vi "Printer Error Handler.vi"(8 "에러 입력(에러 없음)":errorcluster, 10 "큐 데이터":string, 11 "상태":T1 caption="상태 입력") -> (0 "에러 출력":errorcluster, 3 "다음 상태":T1)   [LabVIEW 2010]
doc: "이 템플릿을 사용하여 SubVI로 사용할 VI를 만듭니다."
uses:
  Print Processing States.ctl
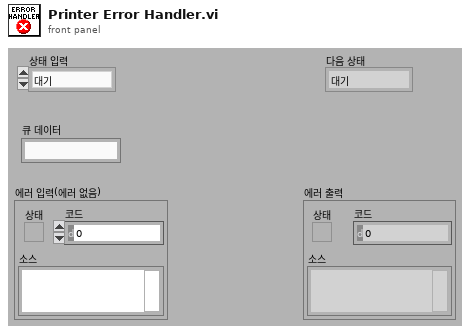
[diagram p1: front panel]
types:
  T1 = typedef "Print Processing States.ctl" = enum16{"대기", "셋업 초기화", "셋업", "인쇄 초기화", "인쇄", "종료"}
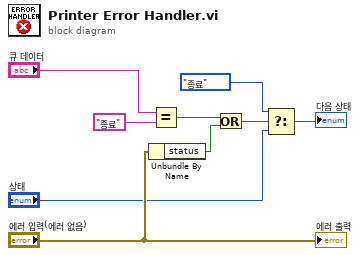
[diagram p0: block diagram]
diagram:
  n1 = Unbundle By Name("에러 입력(에러 없음)") -> ("status"=w6:bool)
  n2 = Equal?(x="큐 데이터", y="종료") -> (x = y?=w5:bool)
  n3 = Or(x=w5, y=w6) -> (x .or. y?=w4:bool)
  n4 = Select(t=Print_Processing_States."종료", s=w4, f="상태") -> (s? t:f=→"다음 상태":T1)
  "에러 출력" <- "에러 입력(에러 없음)"
